vi "Read AI channel.vi"(8 "error in":errorcluster, 11 "analog input mode in":refnum<class "Analog Input Mode.lvclass">) -> (0 "error out":errorcluster, 2 "AI channel":refnum<class "AI Channel.lvclass">, 3 "analog input mode out":refnum<class "Analog Input Mode.lvclass">)   [LabVIEW 2017, in "Scan Engine Scripting.lvlib" / "Analog Input Mode.lvclass"]
doc: "Reads the analog input channel class that is stored in the private data of the analog input mode."
uses:
  Analog Input Vrms Mode/Analog Input Mode.lvclass
  Channel Classes/AI Channel/AI Channel.lvclass
  Analog Input Vrms Mode/Analog Input Mode.lvclass/Analog Input Mode.ctl
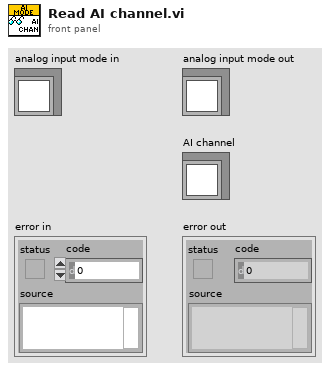
[diagram p1: front panel]
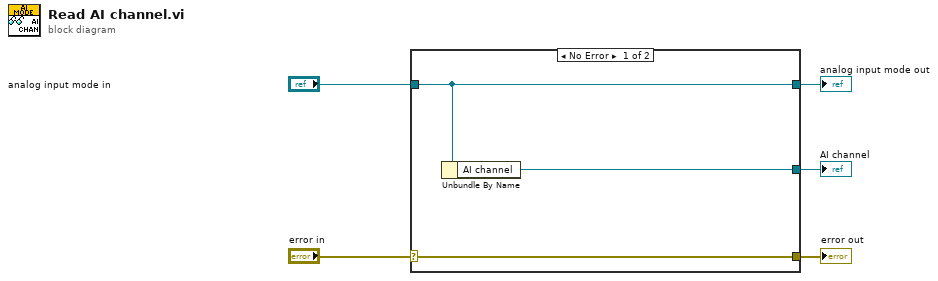
[diagram p0: block diagram]
diagram:
  n1 = case shown="No Error" "error in" {
    selector: "error in" -> [w8 w9]
    tunnel: [w8 w9] -> w4
    tunnel: [w7 w10] -> w2
    tunnel: "analog input mode in" -> [w7 w10]
    tunnel: [w6 _] -> w1
    frame No Error {
      n2 = Unbundle By Name(w7) -> ("AI channel"=w6:refnum<class "AI Channel.lvclass">)
    }
    frame Error {
    }
  }
  "error out" <- w4
  "analog input mode out" <- w2
  "AI channel" <- w1
